vi "SigSyn-Get Valid Sequence Variables.vi"(11 "Stimulus Channel (Full)":T2 caption="Stimulus" {"Filter"."Stages"."IIR Filter"."Forward Coefficients" format="%.4f"; "Filter"."Stages"."IIR Filter"."Reverse Coefficients" format="%.4f"}) -> (3 "Valid Params":string[](array[string]))   [LabVIEW 2015]
uses:
  Controls/Stimulus Channel (Full)/Full Stimulus Channel Data.ctl
  Controls/Waveform XCtl/Waveform Data.ctl
  Controls/Waveform XCtl/Waveform Enum.ctl
  Waveform VIs/Tone VIs/Tone Params.ctl
  Waveform VIs/Pulse Train VIs/Pulse Train Params.ctl
  Waveform VIs/Pulse Train VIs/Pulse Polarity.ctl
  Waveform VIs/Pulse Train VIs/PT-Continuous State.ctl
  Waveform VIs/Noise VIs/Noise Params.ctl
  Waveform VIs/File VIs/StimFile-Params.ctl
  Waveform VIs/FM Sweep VIs/FM Sweep Params.ctl
  Waveform VIs/Chirp Train VIs/Chirp Train.ctl
  Waveform VIs/Chirp Train VIs/Chirp Train Params.ctl
  Waveform VIs/Complex Tone VIs/CT-Params.ctl
  Waveform VIs/Complex Tone VIs/CT-Phase Enum.ctl
  Waveform VIs/Complex Tone VIs/CT-Runtime Data.ctl
  Waveform VIs/Moving Ripple VIs/Moving Ripple.ctl
  Waveform VIs/Moving Ripple VIs/Moving Ripple.Params.ctl
  Waveform VIs/Moving Ripple VIs/Moving Ripple.Data.ctl
  Controls/Advanced Filter XCtl/Filter Data.ctl
  Filter VIs/Filter-Bandwidth Units.ctl
  Controls/Burst XCtl/Burst Data.ctl
  Controls/Level XCtl/Level Data.ctl
  Controls/Level XCtl/Level Units.ctl
  Controls/Advanced Options XCtl/Advanced Stimulus Options.ctl
  Modulation VIs/SAM VIs/SAM Params.ctl
  3rd Generation/XControls/Level (G3)/Level Units (G3).ctl
  3rd Generation/XControls/Level (G3)/Level (G3).xctl
  Controls/Advanced Filter XCtl/Advanced Filter XCtl.xctl
  Controls/Level XCtl/Level XCtl.xctl
  Controls/Burst XCtl/Burst Control.xctl
  Controls/Waveform XCtl/Waveform XCtl.xctl
  Controls/Advanced Options XCtl/Advanced Stimulus Options.xctl
  Controls/Stimulus Channel (Full)/Stimulus Channel (Full).xctl
panel:
  in  "Level.Units":T1
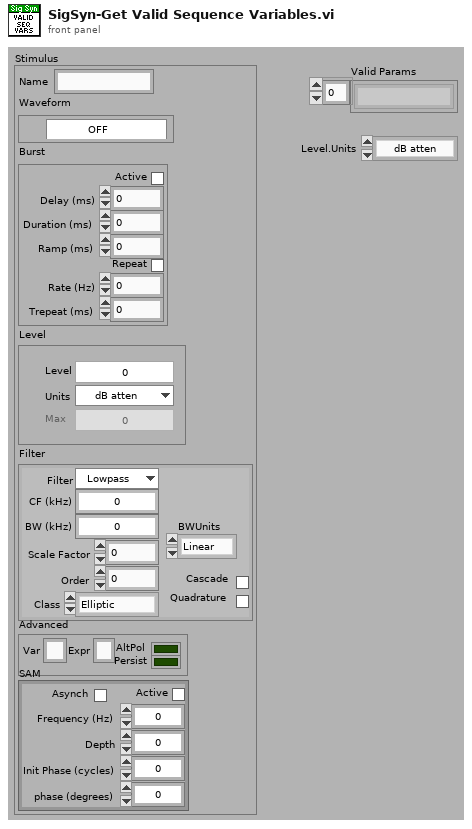
[diagram p1: front panel]
types:
  T1 = typedef "Level (G3).xctl/Level Units (G3).ctl" = enum16{"dB atten", "dB SPL", "dB re 1 Vrms", "dB V/Hz½", "mW", "dB HL", "Volts", "dB mW"}
  T2 = typedef "Stimulus Channel (Full).xctl/Full Stimulus Channel Data.ctl" = cluster{"Waveform":T3, "Filter":T20, "Burst":T22, "Level":T23, "Name":string, "Advanced":T25, "SAM":T26}
  T3 = typedef "Waveform XCtl.xctl/Waveform Data.ctl" = cluster{"Type":T4, "Tone":T5, "Pulse Train":T6, "Noise":T9, "File":T10, "FMSweep":T11, "Chirp Train":T12, "Complex Tone":cluster{"Params":T14, "Data":T16}, "Moving Ripple":T17}
  T4 = typedef "Waveform Enum.ctl" = enum16{"OFF", "Tone", "Noise", "Pulse Train", "File", "FM Sweep", "Chirp Train", "Complex Tone", "FM Tone", "Moving Ripple"}
  T5 = typedef "Tone Params.ctl" = cluster{"Frequency (kHz)":dbl, "Last Freq":dbl, "Last Phase":dbl}
  T6 = typedef "Pulse Train Params.ctl" = cluster{"Pulse width (us)":dbl, "Pulse rate (Hz)":dbl, "Gap (ms)":dbl, "Polarity":T7, "PT State":T8, "Asynch":bool}
  T7 = typedef "Pulse Polarity.ctl" = enum16{"POS", "NEG", "POS-NEG", "NEG-POS"}
  T8 = typedef "PT-Continuous State.ctl" = cluster{"Template":dbl[], "Nperiod":i32, "Index":i32, "Pulse Rate (Hz)":dbl, "Phase (cycles)":dbl, "Noff":i32}
  T9 = typedef "Noise Params.ctl" = cluster{"InvFilt":bool, "Noise":dbl[], "CurPt":i32, "Aweight":bool, "Seed":i32, "afile":path}
  T10 = typedef "StimFile-Params.ctl" = cluster{"Filename":path, "Signal":dbl[], "Channel":i32, "stream":bool, "offset":i32, "nreps":i32, "loops":i32}
  T11 = typedef "FM Sweep Params.ctl" = cluster{"Rate (oct/s)":dbl, "Fmin (Hz)":dbl, "Fmax (Hz)":dbl, "Ramp (ms)":dbl, "Linear":bool}
  T12 = typedef "Chirp Train.ctl" = cluster{"Params":T13, "Data":cluster{"WF":dbl[]}}
  T13 = typedef "Chirp Train Params.ctl" = cluster{"Fmin (kHz)":dbl, "Fmax (kHz)":dbl, "Compensate":bool, "Duration (ms)":dbl}
  T14 = typedef "CT-Params.ctl" = cluster{"F0 (Hz)":dbl, "Band":cluster{"Flow (Hz)":dbl, "Fhigh (Hz)":dbl}, "Phase":T15, "Min F0 (Hz)":dbl, "Max F0 (Hz)":dbl, "ContinRandPhase":bool, "Max peak factor":dbl, "Max mod depth":dbl, "MinHarmNum":i32, "MaxHarmNum":i32, "Level Mode":enum16{"per component", "overall rms"}, "% jitter":dbl}
  T15 = typedef "CT-Phase Enum.ctl" = enum16{"Cosine", "Random", "Alternating"}
  T16 = typedef "CT-Runtime Data.ctl" = cluster{"Ncomp":i32, "MinHarm":i32, "Phase":dbl[], "Amplitude":dbl[], "Npts/frame":i32, "Last F0":dbl, "Fmin":dbl, "Fmax":dbl, "Lslope":dbl, "randphase":bool, "overall rms":bool, "fmult":dbl[], "jittered":bool}
  T17 = typedef "Moving Ripple.ctl" = cluster{"Params":T18, "Data":T19}
  T18 = typedef "Moving Ripple.Params.ctl" = cluster{"Fmin":dbl, "Fmax":dbl, "Density":dbl, "Velocity":dbl, "Depth":dbl, "Phase":dbl, "Comp/oct":i32}
  T19 = typedef "Moving Ripple.Data.ctl" = cluster{"Freq":dbl[], "A":dbl[], "phase":dbl[], "Phase":dbl}
  T20 = typedef "Advanced Filter XCtl.xctl/Filter Data.ctl" = cluster{"Type":enum16{"Lowpass", "Highpass", "Bandpass", "Bandstop", "OFF"}, "CF (kHz)":dbl, "BW (kHz)":dbl, "Cascade":bool, "Quadrature":bool, "Scale Factor":dbl, "Stages":cluster{"IIR Filter":cluster{"filter structure":enum32{"IIR 2nd Order", "IIR 4th Order"}, "Reverse Coefficients":dbl[], "Forward Coefficients":dbl[]}, "State":dbl[]}[], "Class":enum16{"Elliptic", "Butterworth"}, "Order":i32, "BWUnits":T21}
  T21 = typedef "Filter-Bandwidth Units.ctl" = enum16{"Linear", "Octaves", "Min-Max"}
  T22 = typedef "Burst Control.xctl/Burst Data.ctl" = cluster{"Active":bool, "Delay (ms)":dbl, "Duration (ms)":dbl, "Ramp (ms)":dbl, "Rate (Hz)":dbl, "Trepeat (ms)":dbl, "Repeat":bool}
  T23 = typedef "Level XCtl.xctl/Level Data.ctl" = cluster{"Level":dbl, "Units":T24, "Max":dbl, "Multiplier":dbl, "Cal File":path, "Cal":cluster{"Freq (Hz)":dbl[], "Mag (dB SPL)":dbl[], "Phase (deg)":dbl[]}}
  T24 = typedef "Level Units.ctl" = enum16{"dB atten", "dB SPL", "dB re 1 Vrms", "dB V/Hz½", "mW", "dB HL", "Volts", "dB mW"}
  T25 = typedef "Advanced Stimulus Options.xctl/Advanced Stimulus Options.ctl" = cluster{"Rep Mask":string, "AltPol":bool, "Var":string, "Expr":string, "Persist":bool}
  T26 = typedef "SAM Params.ctl" = cluster{"Active":bool, "Frequency (Hz)":dbl, "Depth":dbl, "Init Phase (cycles)":dbl, "phase (degrees)":dbl, "Asynch":bool}
  T27 = enum16{"Lowpass", "Highpass", "Bandpass", "Bandstop", "OFF"}
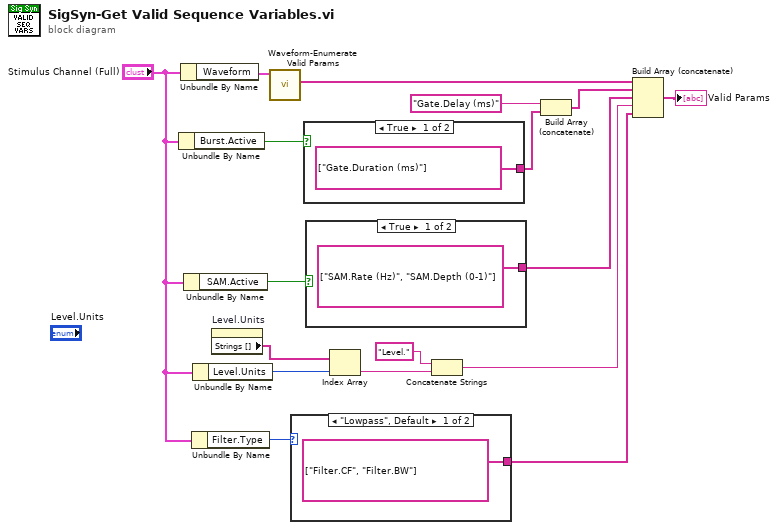
[diagram p0: block diagram]
diagram:
  n1 = Unbundle By Name("Stimulus Channel (Full)") -> ("Burst.Active"=w12:bool)
  n2 = Unbundle By Name("Stimulus Channel (Full)") -> ("Waveform"=w14:T3)
  n3 = Unbundle By Name("Stimulus Channel (Full)") -> ("SAM.Active"=w17:bool)
  n4 = Unbundle By Name("Stimulus Channel (Full)") -> ("Filter.Type"=w8:T27)
  n5 = Unbundle By Name("Stimulus Channel (Full)") -> ("Level.Units"=w4:T24)
  n6 = property on="Level.Units" class="Enum (strict)"() -> ("Strings []"=w5:string[])  [unwired: 2 in, 2 out]
  n7 = call "Waveform-Enumerate Valid Params.vi"("Waveform"=w14) -> ("Parameter Names"=w13:string[])  [unwired: 9 in, 1 out]
  n8 = case shown="\"Lowpass\", Default" w8 {
    tunnel: [string[] ["Filter.CF", "Filter.BW"] _] -> w7
    frame "Lowpass", Default {
    }
    frame "OFF" {
    }
  }
  n9 = case shown="True" w12 {
    tunnel: [string[] ["Gate.Duration (ms)"] _] -> w10
    frame True {
    }
    frame False {
    }
  }
  n10 = case shown="True" w17 {
    tunnel: [string[] ["SAM.Rate (Hz)", "SAM.Depth (0-1)"] _] -> w16
    frame True {
    }
    frame False {
    }
  }
  n11 = Index Array(array=w5, index=w4) -> (element=w3:string)
  n12 = Concatenate Strings("Level.", w3) -> (w1:string)
  n13 = Build Array (concatenate)("Gate.Delay (ms)", w10) -> (w9:string[])
  n14 = Build Array (concatenate)(w13, w9, w16, w1, w7) -> (→"Valid Params":string[])
